vi "Load Input Image.vi"(7 "Path":path, 8 "error in (no error)":errorcluster, 11 "Images":T1) -> (0 "error out":errorcluster, 3 "Images":T1)   [LabVIEW 2015]
uses:
  controls/Images.ctl
  <vilib>/vision/Image Controls.llb/IMAQ Image.ctl
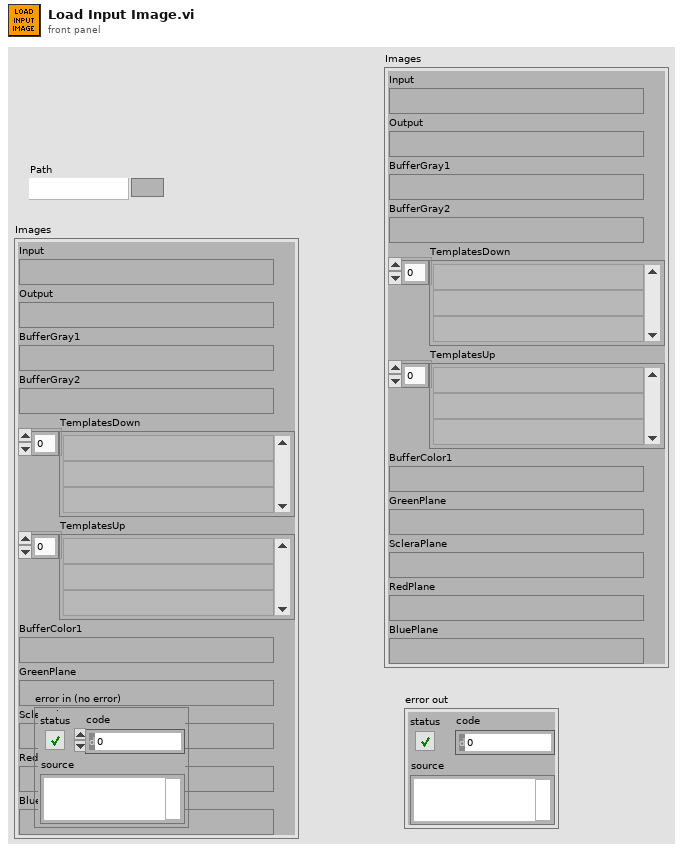
[diagram p1: front panel]
types:
  T1 = typedef "Images.ctl" = cluster{"Input":T2, "Output":T2, "BufferGray1":T2, "BufferGray2":T2, "TemplatesDown":T2[], "TemplatesUp":T2[], "BufferColor1":T2, "GreenPlane":T2, "ScleraPlane":T2, "RedPlane":T2, "BluePlane":T2}
  T2 = typedef "IMAQ Image.ctl" = refnum<image>
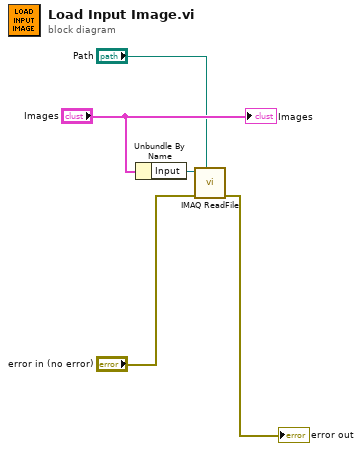
[diagram p0: block diagram]
diagram:
  n1 = Unbundle By Name("Images") -> ("Input"=w5:T2)
  n2 = call "IMAQ ReadFile"("File Path"="Path", "error in (no error)"="error in (no error)", "Image"=w5) -> ("error out"=→"error out":errorcluster)  [unwired: 4 in, 4 out]
  "Images" <- "Images"
